vi "State Exit Core.vi"(8 "error in (no error)":errorcluster, 11 "A Context State in":refnum<class "A Context State.lvclass">) -> (0 "error out":errorcluster, 3 "A Context State out":refnum<class "A Context State.lvclass">)   [LabVIEW 2021, in "Context.lvlib" / "A Context State.lvclass"]
uses:
  A Context State.lvclass
  Context/Context.lvclass
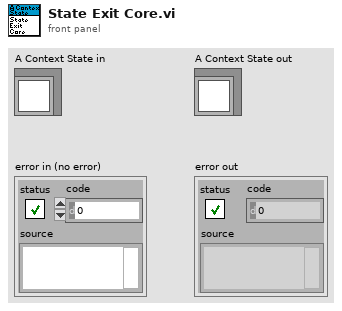
[diagram p1: front panel]
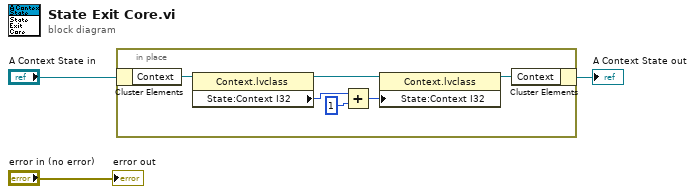
[diagram p0: block diagram]
diagram:
  n1 = in-place {
    n2 = in-place-cluster #1("A Context State in") -> ("Context"=w9:refnum<class "Context.lvclass">)
    n3 = property class="Context.lvclass"(reference=w9) -> (reference out=w8:refnum<class "Context.lvclass">, "State:Context I32"=w6:i32)  [unwired: 1 in, 1 out]
    n4 = Add(x=w6, y=1) -> (x+y=w5:i32)
    n5 = property class="Context.lvclass"(reference=w8, "State:Context I32"=w5) -> (reference out=w7:refnum<class "Context.lvclass">)  [unwired: 1 in, 1 out]
    n6 = in-place-cluster #1("Context"=w7) -> (→"A Context State out":refnum<class "A Context State.lvclass">)
  }
  "error out" <- "error in (no error)"
